vi "Configure Runt Trigger Source [RT] Core.vi"(0 "CS++Scope":refnum<class "CS++Scope.lvclass">, 5 "trigger source (\"CHANNEL1\")":string(combo)="CHANNEL1", 7 "runt low threshold (1.0 V)":dbl[unit]=1.0 format="%.3f", 9 "runt high threshold (4.0 V)":dbl[unit]=4.0 format="%.3f", 11 "error in (no error)":errorcluster) -> (4 "CS++Scope out":refnum<class "CS++Scope.lvclass">, 15 "error out":errorcluster)   [LabVIEW 2015, in "CS++Scope.lvlib" / "CS++Scope.lvclass"]
doc: "This VI configures the runt trigger. A runt trigger occurs when the trigger signal you specify with the Runt Trigger Source parameter crosses one of the runt thresholds twice without crossing the other runt threshold. You specify the runt thresholds with the Runt Low Threshold and Runt High Threshold parameters. You specify the polarity of the runt with the Runt Polarity parameter.\n\nNote \n(1) This VI affects instrument behavior only if the trigger type is\n IVISCOPE_VAL_RUNT_TRIGGER. Call the IviScope Configure Trigger\n and IviScope Configure Trigger Coupling VIs to set the trigger type and\n trigger coupling before calling this VI.\n\n(2) This VI is part of the IviScopeRuntTrigger [RT] extension group."
uses:
  CS++Scope.lvclass
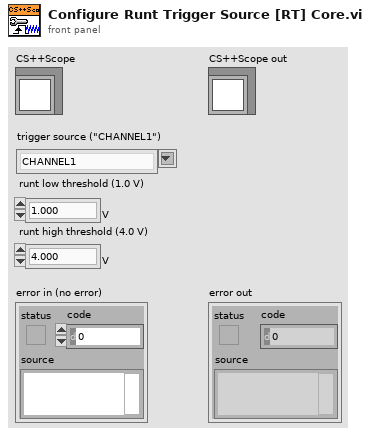
[diagram p1: front panel]
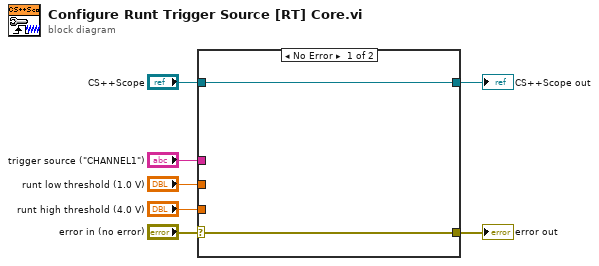
[diagram p0: block diagram]
diagram:
  n1 = case shown="No Error" "error in (no error)" {
    selector: "error in (no error)" -> [w8 w11]
    tunnel: [w8 w11] -> w6
    tunnel: [w9 w10] -> w2
    tunnel: "CS++Scope" -> [w9 w10]
    tunnel: "trigger source (\"CHANNEL1\")" -> [_ _]
    tunnel: "runt low threshold (1.0 V)" -> [_ _]
    tunnel: "runt high threshold (4.0 V)" -> [_ _]
    frame No Error {
    }
    frame Error {
    }
  }
  "error out" <- w6
  "CS++Scope out" <- w2
